vi "Multicolumn Listbox.vi"() -> ()   [LabVIEW 2014]
uses:
  <vilib>/Utility/file.llb/Read From Spreadsheet File (string).vi
panel:
  in  "Multicolumn Listbox 2":i32[](listbox)
  in  "Next Button":bool
  in  "stop":bool
  out "size(s)":i32[](array[numeric])
  in  "Multicolumn Listbox":i32[](listbox)
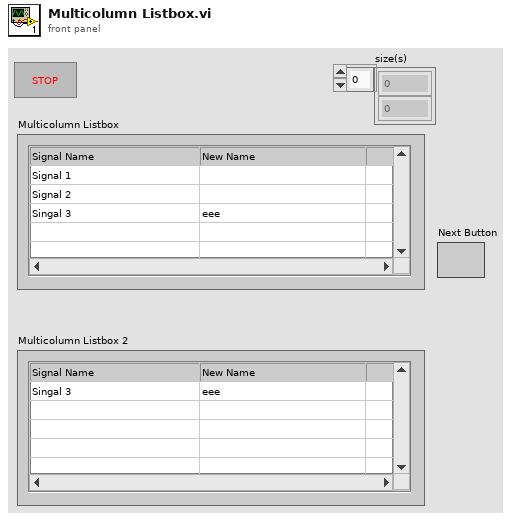
[diagram p1: front panel]
types:
  T1 = typedef "LVPoint32TypeDef.ctl" = cluster{"Horizontal":i32, "Vertical":i32}
  T2 = typedef "LVRowAndColumnTypeDef.ctl" = cluster{"Row":i32, "Column":i32}
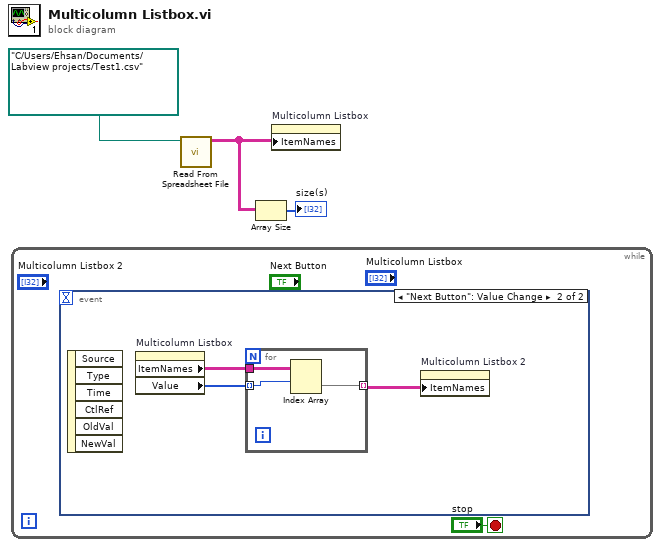
[diagram p0: block diagram]
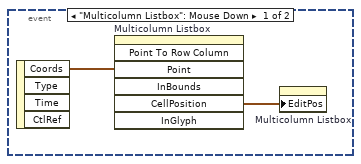
[diagram p2: hidden frame]
diagram:
  n1 = while {
    stop <- "stop" stop-if-true
    n2 = event shown="[1] \"Next Button\": Value Change" {
      selector: _ -> [_ _]
      dyn-events: _ -> [_ _]
      timeout: _ -> [_ _]
      event "Multicolumn Listbox": Mouse Down {
        n3 = event-data() -> ("Coords"=w6:T1)  [unwired: 1 in, 3 out]
        n4 = invoke on="Multicolumn Listbox" class="MCListbox (strict)" method="Point To Row Column"("Point"=w6) -> ("CellPosition"=w5:T2)  [unwired: 6 in, 6 out]
        n5 = property on="Multicolumn Listbox" class="MCListbox (strict)"("EditPos"=w5) -> ()  [unwired: 2 in, 2 out]
      }
      event "Next Button": Value Change {
        n6 = event-data() -> ()  [unwired: 1 in, 6 out]
        n7 = property on="Multicolumn Listbox" class="MCListbox (strict)"() -> ("ItemNames"=w9:string[][], "Value"=w8:i32[])  [unwired: 2 in, 2 out]
        n8 = for {
          tunnel: w9 -> [w12]
          tunnel: w8 -> [w11] mode=indexing
          tunnel: [w10] -> w7 mode=indexing
          n9 = Index Array(array=w12, index (row)=w11) -> (element=w10:string[])  [unwired: 1 in]
        }
        n10 = property on="Multicolumn Listbox 2" class="MCListbox (strict)"("ItemNames"=w7) -> ()  [unwired: 2 in, 2 out]
      }
    }
  }
  n11 = call-poly <vilib>:"Read From Spreadsheet File.vi"("file path (dialog if empty)"=path "C:/Users/Ehsan/Documents/Labview projects/Test1.csv") -> ("all rows"=w2:string[][])  [unwired: 6 in, 4 out]
  n12 = Array Size(array=w2) -> (size(s)=→"size(s)":i32[])
  n13 = property on="Multicolumn Listbox" class="MCListbox (strict)"("ItemNames"=w2) -> ()  [unwired: 2 in, 2 out]
